vi "Splash Screen.vi"(8 "Error In":errorcluster) -> (0 "Error Out":errorcluster, 3 "Status":string)   [LabVIEW 2020]
doc: "This VI check for licensing and load Main program depending on license type."
uses:
  Control/State - Splash Screen.ctl
  Control/Page List Configuration.ctl
  <vilib>/Utility/sysdir.llb/System Directory Type.ctl
  <vilib>/Utility/miscctls.llb/LVPositionTypeDef.ctl
  <vilib>/picture/picture.llb/imagedata.ctl
  Control/License File Parameter.ctl
panel:
  in  "EXE Name":string="VSys Platform"
  out "Computer ID":string
  in  "stop":bool
  out "Version":string
  out "BG Image":picture
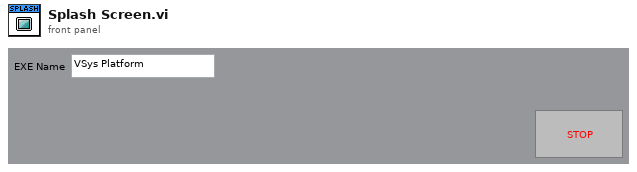
[diagram p1: front panel]
types:
  T1 = typedef "Page List Configuration.ctl" = cluster{"HMI Configuration":cluster{"EXE Name":string, "Project Name":string, "Max Page No":i32, "HMI State":enum32{"Invalid", "Standard", "Closed", "Hidden", "Minimized", "Maximized"}, "Version":enum16{"Demo", "User"}, "Check License":bool, "Font Size":u32, "Res: Height":i16, "Res: Width":i16, "License Level":enum16{"Level 1", "Level 2", "Level 3", "Level 4", "Level 5"}, "License Type":enum16{"Free", "Trial", "Subscription", "Perpetual"}}, "All HMI Module":string[], "Default HMI Module":string[], "Page Module":string[], "Page List: Level 1":string[], "Page List: Level 2":string[], "Page List: Level 3":string[], "All RT Module":string[], "Default RT Module":string[], "Acquire Enable Page":string[], "Log Enable Page":string[], "Run Page":string[], "Kill Page":string[], "Button":cluster{"Text":string[], "Tip Strip":string[]}}
  T2 = typedef "State - Splash Screen.ctl" = enum16{"Init", "Read Config", "Set BG Image", "Get Computer ID", "Check Licensing", "Load Main VI", "Close"}
  T3 = enum32{"Invalid", "Standard", "Closed", "Hidden", "Minimized", "Maximized"}
  T4 = typedef "LVPositionTypeDef.ctl" = cluster{"Left":i32, "Top":i32}
  T5 = enum16{"open", "replace", "create", "open or create", "replace or create", "replace or create with confirmation"}
  T6 = typedef "imagedata.ctl" = cluster{"image type":i32, "image depth":i32, "image":u8[], "mask":u8[], "colors":u32[], "Rectangle":cluster{"left":i16, "top":i16, "right":i16, "bottom":i16}}
  T7 = enum16{"Level 1", "Level 2", "Level 3", "Level 4", "Level 5"}
  T8 = typedef "License File Parameter.ctl" = cluster{"Expired Time":string, "Computer ID":string, "Product Name":string, "Period":i16, "Activated Time":string, "License Level":enum16{"Level 1", "Level 2", "Level 3", "Level 4", "Level 5"}, "License Type":enum16{"Free", "Trial", "Subscription", "Perpetual"}, "Log Time":string}
  T9 = enum32{"invalid app kind", "Development System", "Run Time System", "Student Edition", "Embedded LabVIEW", "Evaluation", "Custom"}
  T10 = typedef "System Directory Type.ctl" = i32
  T11 = enum16{"Free", "Trial", "Subscription", "Perpetual"}
  T12 = enum32{"Bad", "Idle", "Run top level", "Running"}
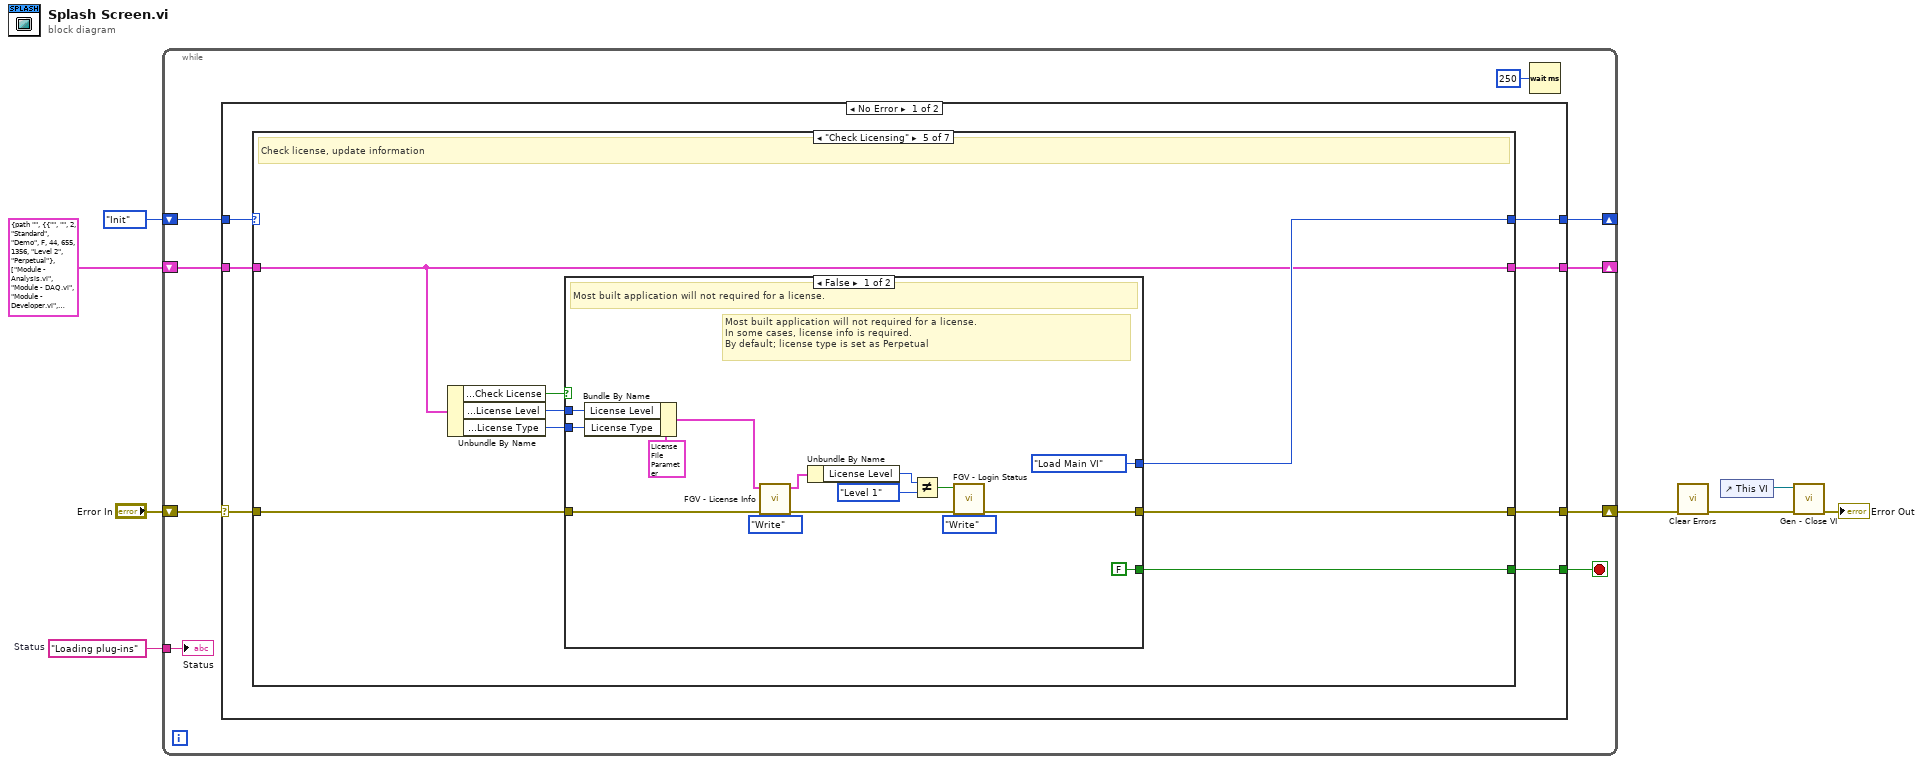
[diagram p0: block diagram]
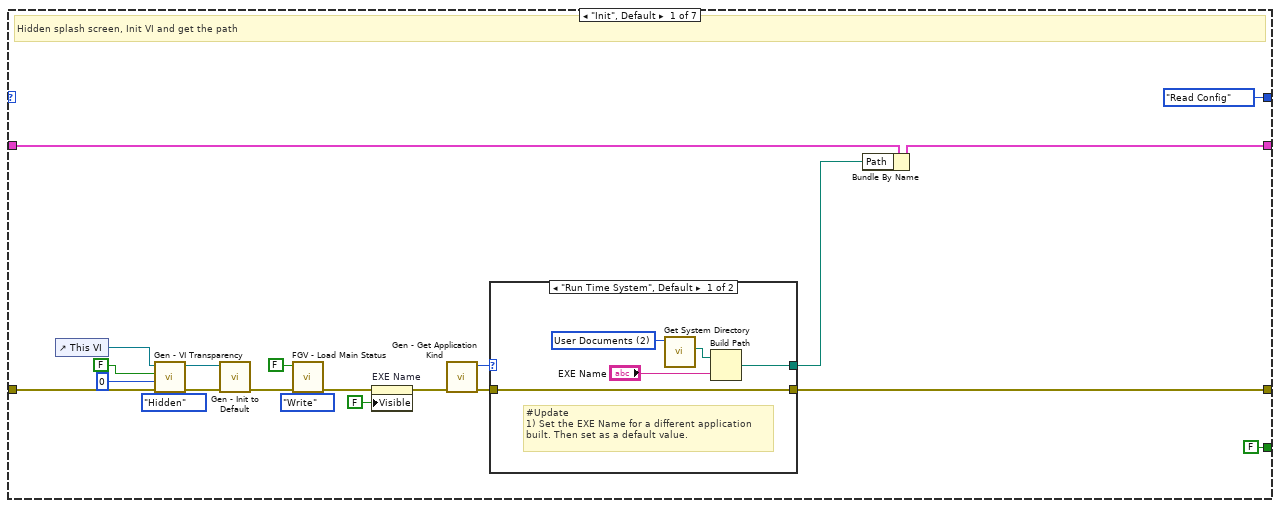
[diagram p2: hidden frame]
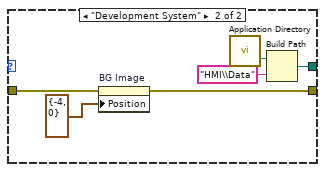
[diagram p3: hidden frame]
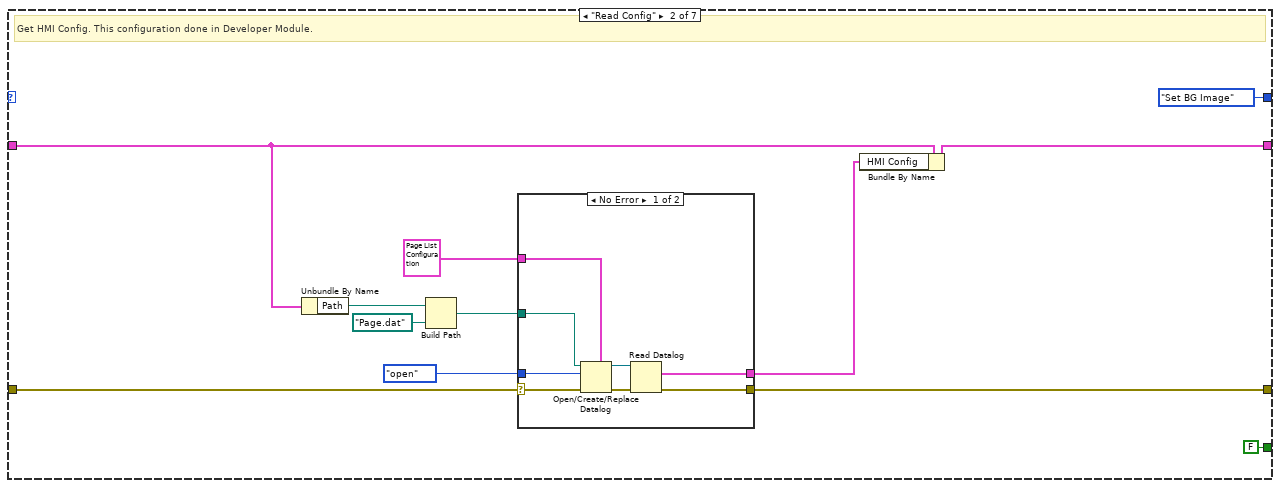
[diagram p4: hidden frame]
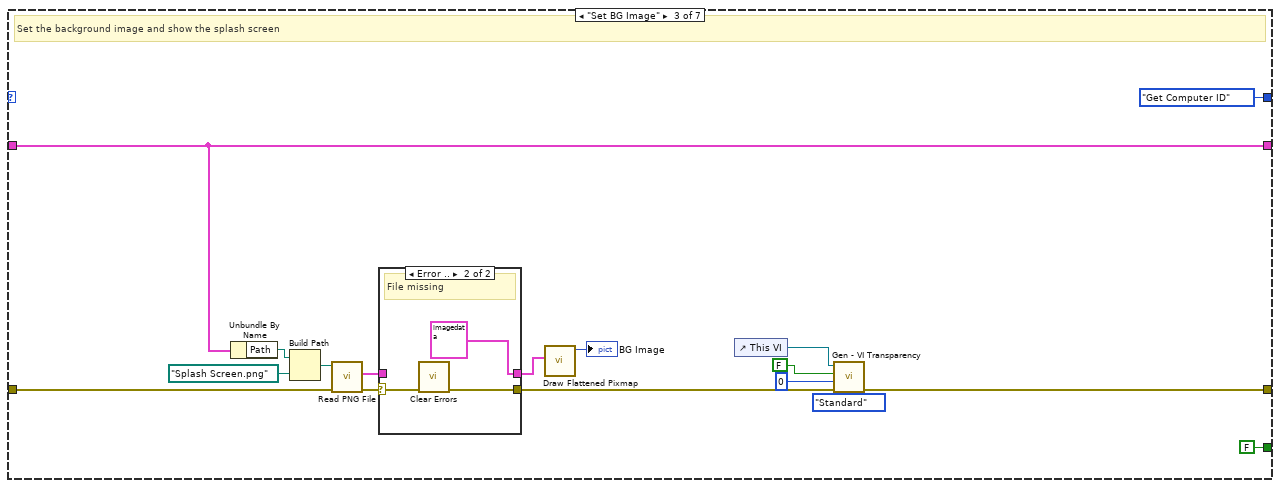
[diagram p6: hidden frame]
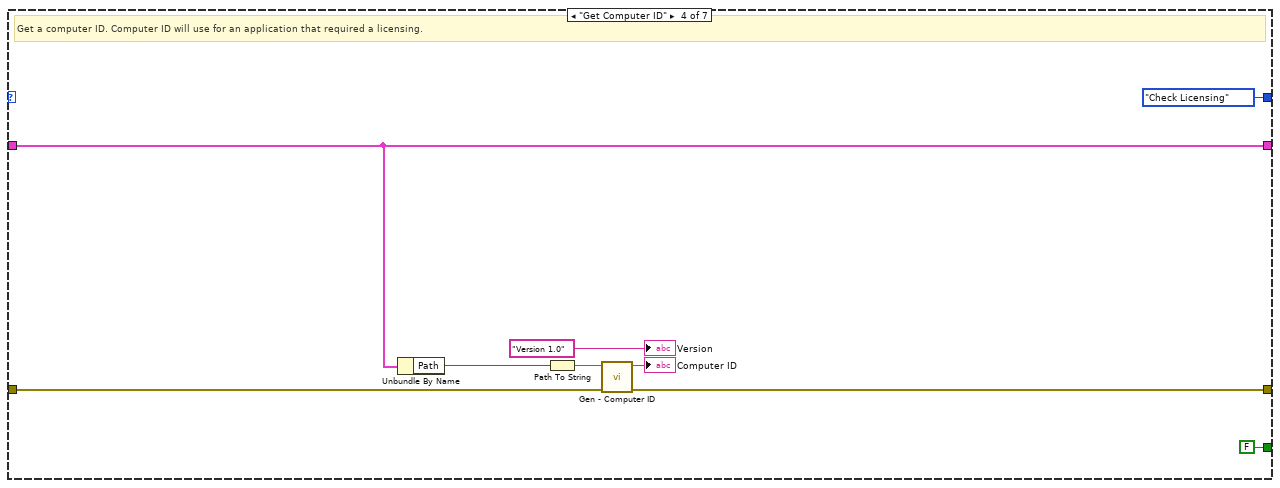
[diagram p8: hidden frame]
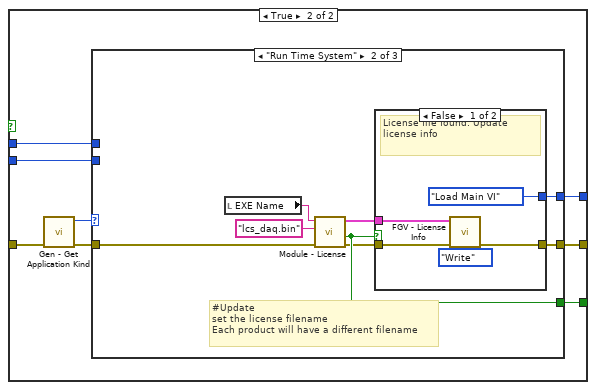
[diagram p9: hidden frame]
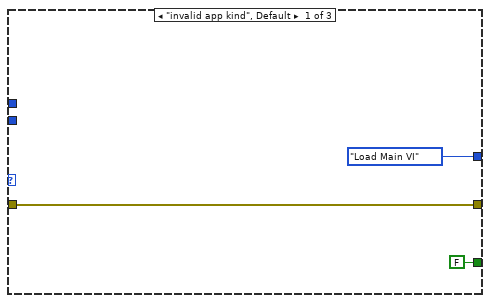
[diagram p10: hidden frame]
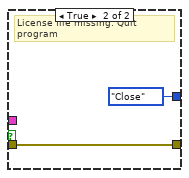
[diagram p11: hidden frame]
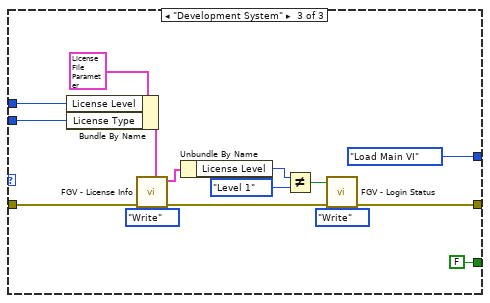
[diagram p12: hidden frame]
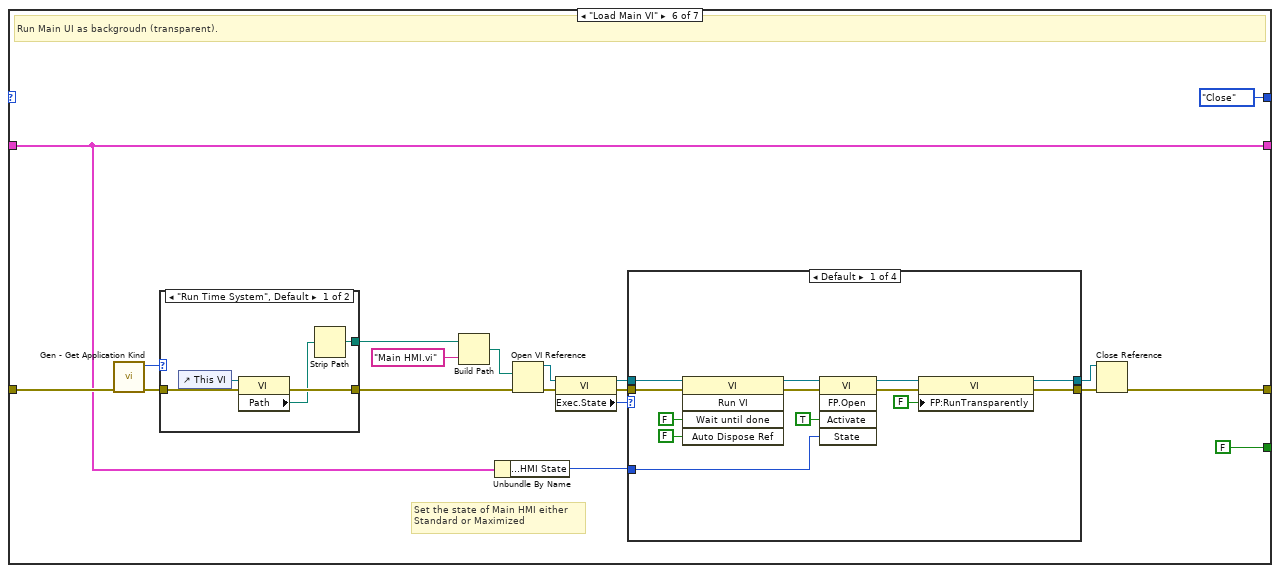
[diagram p13: hidden frame]
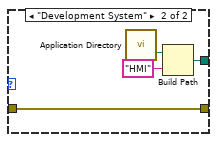
[diagram p14: hidden frame]
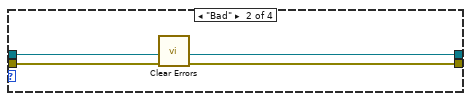
[diagram p15: hidden frame]
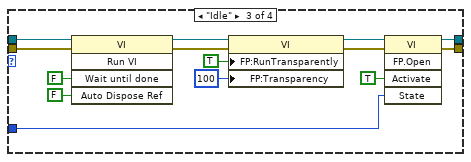
[diagram p16: hidden frame]
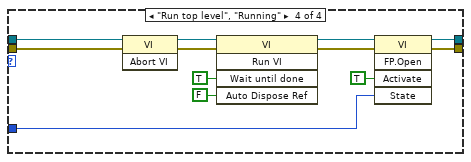
[diagram p17: hidden frame]
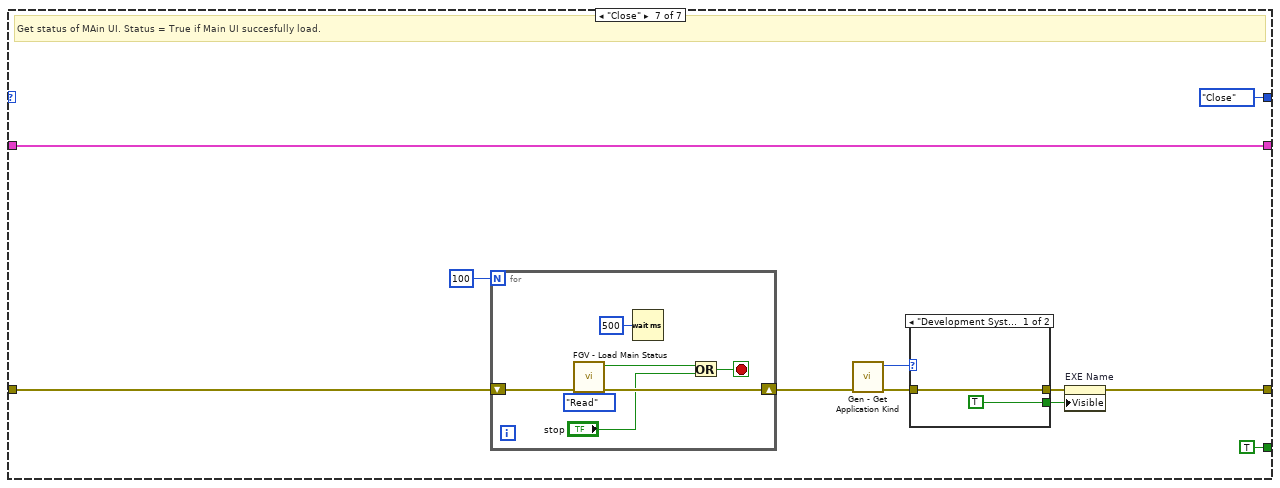
[diagram p18: hidden frame]
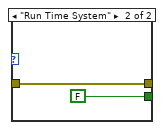
[diagram p19: hidden frame]
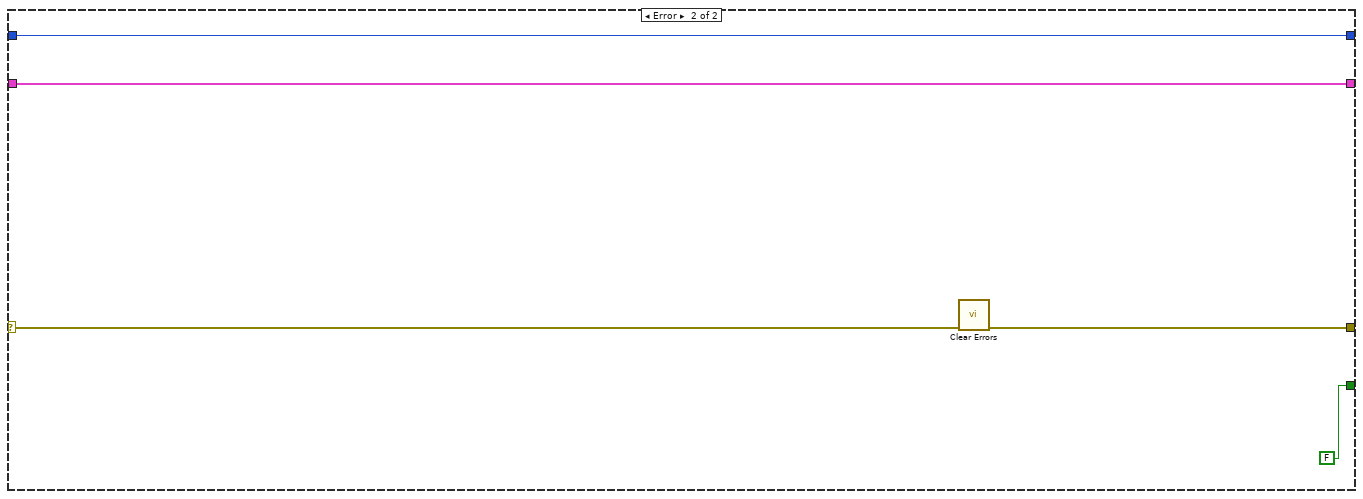
[diagram p20: hidden frame]
diagram:
  w7 = "Loading plug-ins"  # Status
  n1 = while {
    shift-right: [w16] -> w5
    shift-left: "Error In" -> [w17]
    shift-right: [w13] -> _
    shift-left: State_-_Splash_Screen."Init" ("State") -> [w15]
    tunnel: w7 -> [w11]
    shift-right: [w9] -> _
    shift-left: cluster{"Path":path, "HMI Config":T1} {"Path"=path "", "HMI Config"={"HMI Configuration"={"EXE Name"="", "Project Name"="", "Max Page No"=2, "HMI State"=enum."Standard", "Version"=enum."Demo", "Check License"=FALSE, "Font Size"=44, "Res: Height"=655, "Res: Width"=1356, "License Level"=enum."Level 2", "License Type"=enum."Perpetual"}, "All HMI Module"=["Module - Analysis.vi", "Module - DAQ.vi", "Module - Developer.vi", "Module - Error Management.vi", "Module - License.vi", "Module - Logging.vi", "Module - Network Stream PC.vi", "Module - NSV Comm PC.vi", "Module - Page Configuration.vi", "Module - Page Main.vi", "Module - Page Prediction.vi", "Module - Page Ranging.vi", "Module - Page User.vi", "Module - Template HMI - Copy.vi", "Module - Template HMI.vi", "Module - WebDAV.vi"], "Default HMI Module"=["Module - DAQ.vi", "Module - Network Stream PC.vi", "Module - NSV Comm PC.vi", "Module - Page Configuration.vi", "Module - Page Ranging.vi", "Module - Page Logging.vi", "Module - Analysis.vi", "Module - Page Prediction.vi"], "Page Module"=["Module - Page Configuration.vi", "Module - Page Ranging.vi", "Module - Analysis.vi", "Module - Page Prediction.vi"], "Page List: Level 1"=["Module - Page Main.vi", "Module - Page Device.vi", "Module - Page IO Setting.vi", "Module - Page Logging.vi", "Module - Page Scale.vi", "Module - Page Filter.vi", "Module - Page User.vi", "Module - Page Cloud.vi"], "Page List: Level 2"=["Module - Page Main.vi", "Module - Page Device.vi", "Module - Page IO Setting.vi", "Module - Page Logging.vi", "Module - Page Scale.vi", "Module - Page Filter.vi"], "Page List: Level 3"=["Module - Page Main.vi", "Module - Page Device.vi", "Module - Page IO Setting.vi"], "All RT Module"=[], "Default RT Module"=["Module - Page Configuration.vi", "Module - Page Main.vi"], "Acquire Enable Page"=["Module - Page Configuration.vi", "Module - Page Ranging.vi"], "Log Enable Page"=["Module - RT Device.vi", "Module - RT Git.vi"], "Run Page"=["Module - DAQmx AI.vi", "Module - DAQmx AO.vi", "Module - DAQmx DI.vi", "Module - DAQmx DO.vi"], "Kill Page"=["Module - Arduino DIO AI.vi"], "Button"={"Text"=["CONFIGURE", "RANGING", "ANALYSIS", "PREDICTION", "SCALE", "FILTER", "USER", "CLOUD", "ALARM", "Button 10", "Button 11", "Button 12", "Button 13", "Button 14", "Button 15"], "Tip Strip"=[]}}} -> [w10]
    stop <- w14 stop-if-true
    n2 = case shown="No Error" w17 {
      selector: w17 -> [w23 w270]
      tunnel: w15 -> [w22 w267]
      tunnel: [w24 w269] -> w16
      tunnel: [w21 FALSE] -> w14
      tunnel: [w20 w267] -> w13
      tunnel: w10 -> [w19 w266]
      tunnel: [w18 w266] -> w9
      frame No Error {
        n3 = case shown="\"Check Licensing\"" w22 {
          tunnel: [w26 w62 w79 w106 w117 w176 w248] -> w24
          tunnel: w23 -> [w41 w59 w90 w107 w114 w180 w254]
          tunnel: [FALSE FALSE FALSE ("License Missing?") FALSE ("License Missing?") w115 FALSE TRUE] -> w21
          tunnel: [State_-_Splash_Screen."Read Config" ("State") State_-_Splash_Screen."Set BG Image" ("State") State_-_Splash_Screen."Get Computer ID" ("State") State_-_Splash_Screen."Check Licensing" ("State") w116 State_-_Splash_Screen."Close" ("State") State_-_Splash_Screen."Close" ("State")] -> w20
          tunnel: w19 -> [w31 w61 w89 w105 w113 w175 w244]
          tunnel: [w27 w58 w89 w105 w113 w175 w244] -> w18
          frame "Init", Default {
            # "Hidden splash screen, Init VI and get the path"
            n4 = control-ref of="This VI"() -> (w43:refnum<vi>)
            n5 = call "Gen - VI Transparency.vi"("State"=T3."Hidden", "Error In"=w41, "Transparency"=u8 0, "Transparently?"=FALSE, "Ref VI"=w43) -> ("Error Out"=w42:errorcluster, "Ref VI Out"=w36:refnum<vi>)  [unwired: 5 in]
            n6 = call "Gen - Init to Default.vi"("Error in"=w42, "This VI"=w36) -> ("Error out"=w35:errorcluster)  [unwired: 8 in, 1 out]
            n7 = call "FGV - Load Main Status.vi"("Action"=enum16{"Read", "Write"}."Write", "Error In"=w35, "Status in"=FALSE) -> ("Error Out"=w33:errorcluster)  [unwired: 7 in, 1 out]
            n8 = property on="EXE Name" class="Str"(error in=w33, "Visible"=FALSE) -> (error out=w28:errorcluster)  [unwired: 1 in, 1 out]
            n9 = call "Gen - Get Application Kind.vi"("Error In"=w28) -> ("Error Out"=w29:errorcluster, "Application:Kind"=w30:T9)  [unwired: 9 in]
            n10 = case shown="\"Run Time System\", Default" w30 {
              tunnel: [w46 w54] -> w25
              tunnel: [w50 w52] -> w26
              tunnel: w29 -> [w50 w53]
              frame "Run Time System", Default {
                w47 = T10 2 items=["User Home"=0, "User Desktop"=1, "User Documents"=2, "User Application Data"=3, "User Preferences"=4, "User Temporary"=5, "Public Documents"=6, "Public Application Data"=7, "Public Preferences"=8, "Public Cache"=13, "System Core Libraries"=9, "System Installed Libraries"=10, "Application Files"=11, "Boot Volume Root"=12] ("system directory type")
                # "#Update\n1) Set the EXE Name for a different application \nbuilt. Then set as a default value."
                n11 = call <vilib>:"Get System Directory.vi"("system directory type"=w47) -> ("system directory"=w49:path)  [unwired: 10 in]
                n12 = Build Path(base path=w49, name or relative path="EXE Name") -> (appended path=w46:path)
              }
              frame "Development System" {
                n13 = property on="BG Image" class="Pict"(error in=w53, "Position"=T4 {"Left"=-4, "Top"=0}) -> (error out=w52:errorcluster)  [unwired: 1 in, 1 out]
                n14 = call <vilib>:"Application Directory.vi"() -> ("Application Directory"=w55:path)
                n15 = Build Path(base path=w55, name or relative path="HMI\\Data") -> (appended path=w54:path)
              }
            }
            n16 = Bundle By Name(cluster=w31, "Path"=w25) -> (w27:cluster{"Path":path, "HMI Config":T1})
          }
          frame "Read Config" {
            # "Get HMI Config. This configuration done in Developer Module."
            n17 = Unbundle By Name(w61) -> ("Path"=w60:path)
            n18 = Build Path(base path=w60, name or relative path=path "Page.dat") -> (appended path=w63:path)
            n19 = case shown="No Error" w59 {
              selector: w59 -> [w70 w78]
              tunnel: T1 {"HMI Configuration"={"EXE Name"="", "Project Name"="", "Max Page No"=2, "HMI State"=enum."Standard", "Version"=enum."Demo", "Check License"=FALSE, "Font Size"=44, "Res: Height"=655, "Res: Width"=1356, "License Level"=enum."Level 2", "License Type"=enum."Perpetual"}, "All HMI Module"=["Module - Analysis.vi", "Module - DAQ.vi", "Module - Developer.vi", "Module - Error Management.vi", "Module - License.vi", "Module - Logging.vi", "Module - Network Stream PC.vi", "Module - NSV Comm PC.vi", "Module - Page Configuration.vi", "Module - Page Main.vi", "Module - Page Prediction.vi", "Module - Page Ranging.vi", "Module - Page User.vi", "Module - Template HMI - Copy.vi", "Module - Template HMI.vi", "Module - WebDAV.vi"], "Default HMI Module"=["Module - DAQ.vi", "Module - Network Stream PC.vi", "Module - NSV Comm PC.vi", "Module - Page Configuration.vi", "Module - Page Ranging.vi", "Module - Page Logging.vi", "Module - Analysis.vi", "Module - Page Prediction.vi"], "Page Module"=["Module - Page Configuration.vi", "Module - Page Ranging.vi", "Module - Analysis.vi", "Module - Page Prediction.vi"], "Page List: Level 1"=["Module - Page Main.vi", "Module - Page Device.vi", "Module - Page IO Setting.vi", "Module - Page Logging.vi", "Module - Page Scale.vi", "Module - Page Filter.vi", "Module - Page User.vi", "Module - Page Cloud.vi"], "Page List: Level 2"=["Module - Page Main.vi", "Module - Page Device.vi", "Module - Page IO Setting.vi", "Module - Page Logging.vi", "Module - Page Scale.vi", "Module - Page Filter.vi"], "Page List: Level 3"=["Module - Page Main.vi", "Module - Page Device.vi", "Module - Page IO Setting.vi"], "All RT Module"=[], "Default RT Module"=["Module - Page Configuration.vi", "Module - Page Main.vi"], "Acquire Enable Page"=["Module - Page Configuration.vi", "Module - Page Ranging.vi"], "Log Enable Page"=["Module - RT Device.vi", "Module - RT Git.vi"], "Run Page"=["Module - DAQmx AI.vi", "Module - DAQmx AO.vi", "Module - DAQmx DI.vi", "Module - DAQmx DO.vi"], "Kill Page"=["Module - Arduino DIO AI.vi"], "Button"={"Text"=["CONFIGURE", "RANGING", "ANALYSIS", "PREDICTION", "SCALE", "FILTER", "USER", "CLOUD", "ALARM", "Button 10", "Button 11", "Button 12", "Button 13", "Button 14", "Button 15"], "Tip Strip"=[]}} ("Data Out 2") -> [w75 w77]
              tunnel: T5."open" ("operation (0:open)") -> [w74 _]
              tunnel: w63 -> [w73 _]
              tunnel: [w71 w78] -> w62
              tunnel: [w69 w77] -> w57
              frame No Error {
                n20 = Open/Create/Replace Datalog(5:w75, 8:w70, 10:w74, 11:w73) -> (0:w72:errorcluster, 3:w76:refnum<k1>)  [unwired: 2 in, 1 out]
                n21 = Read Datalog(4:w72, 7:w76) -> (0:w71:errorcluster, 2:w69:T1)  [unwired: 1 in, 1 out]
              }
              frame Error {
              }
            }
            n22 = Bundle By Name(cluster=w61, "HMI Config"=w57) -> (w58:cluster{"Path":path, "HMI Config":T1})
          }
          frame "Set BG Image" {
            # "Set the background image and show the splash screen"
            n23 = Unbundle By Name(w89) -> ("Path"=w88:path)
            n24 = Build Path(base path=w88, name or relative path=path "Splash Screen.png") -> (appended path=w93:path)
            n25 = call <vilib>:"Read PNG File.vi"("error in (no error)"=w90, "path to PNG file"=w93) -> ("error out"=w87:errorcluster, "image data"=w85:T6)  [unwired: 7 in, 1 out]
            n26 = case shown="Error .." w87 {
              selector: w87 -> [w97 w99]
              tunnel: [w97 w98] -> w86
              tunnel: [w96 T6 {"image type"=0, "image depth"=32, "image"=array[1013796 elements], "mask"=array[32184 elements], "colors"=[], "Rectangle"={"left"=0, "top"=0, "right"=567, "bottom"=447}} ("image data")] -> w84
              tunnel: w85 -> [w96 _]
              frame No Error {
              }
              frame Error {
                # "File missing"
                n27 = call <vilib>:"Clear Errors.vi"("error in (no error)"=w99) -> ("error out"=w98:errorcluster)  [unwired: 5 in, 1 out]
              }
            }
            n28 = call <vilib>:"Draw Flattened Pixmap.vi"("image data"=w84) -> ("new picture"=→"BG Image":picture)  [unwired: 8 in]
            n29 = control-ref of="This VI"() -> (w83:refnum<vi>)
            n30 = call "Gen - VI Transparency.vi"("State"=T3."Standard", "Error In"=w86, "Transparency"=u8 0, "Transparently?"=FALSE, "Ref VI"=w83) -> ("Error Out"=w79:errorcluster)  [unwired: 5 in, 1 out]
          }
          frame "Get Computer ID" {
            # "Get a computer ID. Computer ID will use for an application that required a licensing."
            n31 = Unbundle By Name(w105) -> ("Path"=w104:path)
            n32 = Path To String(path=w104) -> (string=w102:string)
            n33 = call "Gen - Computer ID.vi"("Error In"=w107, "Path"=w102) -> ("Error Out"=w106:errorcluster, "COMPUTER ID"=→"Computer ID":string)  [unwired: 8 in]
            "Version" <- "Version 1.0" ("Serial Number")
          }
          frame "Check Licensing" {
            # "Check license, update information"
            n34 = Unbundle By Name(w113) -> ("HMI Config.HMI Configuration.Check License"=w112:bool, "HMI Config.HMI Configuration.License Level"=w111:T7, "HMI Config.HMI Configuration.License Type"=w110:T11)
            n35 = case shown="False" w112 {
              tunnel: [w123 w140] -> w117
              tunnel: [State_-_Splash_Screen."Load Main VI" ("State") w139] -> w116
              tunnel: [FALSE ("License Missing?") w138] -> w115
              tunnel: w114 -> [w130 w137]
              tunnel: w111 -> [w119 w134]
              tunnel: w110 -> [w118 w133]
              frame False {
                # "Most built application will not required for a license. \nIn some cases, license info is required.\nBy default; license type is set as Perpetual"
                # "Most built application will not required for a license."
                n36 = Bundle By Name(cluster=T8 {"Expired Time"="", "Computer ID"="", "Product Name"="", "Period"=0, "Activated Time"="", "License Level"=enum."Level 1", "License Type"=enum."Perpetual", "Log Time"=""} ("License Info  In"), "License Level"=w119, "License Type"=w118) -> (w120:T8)
                n37 = call "FGV - License Info.vi"("FGV States"=enum16{"Read", "Write"}."Write", "Error In"=w130, "License Info  In"=w120) -> ("Error Out"=w126:errorcluster, "License Info"=w122:T8)  [unwired: 7 in]
                n38 = Unbundle By Name(w122) -> ("License Level"=w125:T7)
                n39 = Not Equal?(x=w125, y=T7."Level 1" ("License Level")) -> (x != y?=w121:bool)
                n40 = call "FGV - Login Status.vi"("Action"=enum16{"Read", "Write"}."Write", "Error In"=w126, "Login In"=w121) -> ("Error Out"=w123:errorcluster)  [unwired: 6 in, 2 out]
              }
              frame True {
                n41 = call "Gen - Get Application Kind.vi"("Error In"=w137) -> ("Error Out"=w136:errorcluster, "Application:Kind"=w135:T9)  [unwired: 9 in]
                n42 = case shown="\"Run Time System\"" w135 {
                  tunnel: w136 -> [w143 w151 w172]
                  tunnel: [w143 w150 w163] -> w140
                  tunnel: [State_-_Splash_Screen."Load Main VI" ("State") w149 State_-_Splash_Screen."Load Main VI" ("State")] -> w139
                  tunnel: [FALSE ("License Missing?") w148 FALSE ("License Missing?")] -> w138
                  tunnel: w134 -> [_ _ w160]
                  tunnel: w133 -> [_ _ w159]
                  frame "invalid app kind", Default {
                  }
                  frame "Run Time System" {
                    # "#Update\nset the license filename\nEach product will have a different filename"
                    n43 = local read "EXE Name"() -> (w144:string)
                    n44 = call "Module - License.vi"("Error In"=w151, "License Filename"="lcs_daq.bin", "Product Name"=w144) -> ("Error Out"=w147:errorcluster, "License Missing?"=w148:bool, "License Info"=w146:T8)  [unwired: 4 in, 2 out]
                    n45 = case shown="False" w148 {
                      tunnel: [w156 w157] -> w150
                      tunnel: [State_-_Splash_Screen."Load Main VI" ("State") State_-_Splash_Screen."Close" ("State")] -> w149
                      tunnel: w147 -> [w153 w157]
                      tunnel: w146 -> [w152 _]
                      frame False {
                        # "License file found. Update license info"
                        n46 = call "FGV - License Info.vi"("FGV States"=enum16{"Read", "Write"}."Write", "Error In"=w153, "License Info  In"=w152) -> ("Error Out"=w156:errorcluster)  [unwired: 7 in, 1 out]
                      }
                      frame True {
                        # "License file missing. Quit program"
                      }
                    }
                  }
                  frame "Development System" {
                    n47 = Bundle By Name(cluster=T8 {"Expired Time"="", "Computer ID"="", "Product Name"="", "Period"=0, "Activated Time"="", "License Level"=enum."Level 2", "License Type"=enum."Perpetual", "Log Time"=""} ("License Info  In"), "License Level"=w160, "License Type"=w159) -> (w161:T8)
                    n48 = call "FGV - License Info.vi"("FGV States"=enum16{"Read", "Write"}."Write", "Error In"=w172, "License Info  In"=w161) -> ("Error Out"=w164:errorcluster, "License Info"=w168:T8)  [unwired: 7 in]
                    n49 = Unbundle By Name(w168) -> ("License Level"=w167:T7)
                    n50 = Not Equal?(x=w167, y=T7."Level 1" ("License Level")) -> (x != y?=w165:bool)
                    n51 = call "FGV - Login Status.vi"("Action"=enum16{"Read", "Write"}."Write", "Error In"=w164, "Login In"=w165) -> ("Error Out"=w163:errorcluster)  [unwired: 6 in, 2 out]
                  }
                }
              }
            }
          }
          frame "Load Main VI" {
            # "Set the state of Main HMI either \nStandard or Maximized"
            # "Run Main UI as backgroudn (transparent)."
            n52 = call "Gen - Get Application Kind.vi"("Error In"=w180) -> ("Error Out"=w179:errorcluster, "Application:Kind"=w181:T9)  [unwired: 9 in]
            n53 = case shown="\"Run Time System\", Default" w181 {
              tunnel: [w193 w198] -> w185
              tunnel: [w196 w201] -> w182
              tunnel: w179 -> [w195 w201]
              frame "Run Time System", Default {
                n54 = control-ref of="This VI"() -> (w197:refnum<vi>)
                n55 = property class="VI"(reference=w197, error in=w195) -> (error out=w196:errorcluster, "Path"=w194:path)  [unwired: 1 out]
                n56 = Strip Path(path=w194) -> (stripped path=w193:path)  [unwired: 1 out]
              }
              frame "Development System" {
                n57 = call <vilib>:"Application Directory.vi"() -> ("Application Directory"=w199:path)
                n58 = Build Path(base path=w199, name or relative path="HMI") -> (appended path=w198:path)
              }
            }
            n59 = Build Path(base path=w185, name or relative path="Main HMI.vi") -> (appended path=w183:path)
            n60 = Unbundle By Name(w175) -> ("HMI Config.HMI Configuration.HMI State"=w174:T3)
            n61 = Open VI Reference(vi path=w183, error in (no error)=w182) -> (vi reference=w188:refnum<vi>, error out=w187:errorcluster)  [unwired: 4 in]
            n62 = property class="VI"(reference=w188, error in=w187) -> (reference out=w190:refnum<vi>, error out=w189:errorcluster, "Exec.State"=w191:T12)
            n63 = case shown="Default" w191 {
              tunnel: w189 -> [w212 w217 w229 w243]
              tunnel: w190 -> [w211 w216 w228 w242]
              tunnel: [w206 w216 w226 w234] -> w178
              tunnel: [w205 w215 w225 w233] -> w177
              tunnel: w174 -> [w202 _ w218 w232]
              frame Default {
                n64 = invoke class="VI" method="Run VI"(reference=w211, error in=w212, "Wait until done"=FALSE ("Wait Until Done"), "Auto Dispose Ref"=FALSE ("Auto Dispose Reference")) -> (reference out=w209:refnum<vi>, error out=w210:errorcluster)  [unwired: 1 in, 3 out]
                n65 = invoke class="VI" method="FP.Open"(reference=w209, error in=w210, "Activate"=TRUE ("Activate?"), "State"=w202) -> (reference out=w207:refnum<vi>, error out=w204:errorcluster)  [unwired: 1 in, 3 out]
                n66 = property class="VI"(reference=w207, error in=w204, "FP:RunTransparently"=FALSE ("Front Panel Window:Run VI Transparently")) -> (reference out=w206:refnum<vi>, error out=w205:errorcluster)
              }
              frame "Bad" {
                n67 = call <vilib>:"Clear Errors.vi"("error in (no error)"=w217) -> ("error out"=w215:errorcluster)  [unwired: 5 in, 1 out]
              }
              frame "Idle" {
                n68 = invoke class="VI" method="Run VI"(reference=w228, error in=w229, "Wait until done"=FALSE ("Wait Until Done"), "Auto Dispose Ref"=FALSE ("Auto Dispose Reference")) -> (reference out=w221:refnum<vi>, error out=w223:errorcluster)  [unwired: 1 in, 3 out]
                n69 = property class="VI"(reference=w221, error in=w223, "FP:RunTransparently"=TRUE ("Front Panel Window:Run VI Transparently"), "FP:Transparency"=u8 100 ("Front Panel Window:Transparency")) -> (reference out=w220:refnum<vi>, error out=w222:errorcluster)
                n70 = invoke class="VI" method="FP.Open"(reference=w220, error in=w222, "Activate"=TRUE ("Activate?"), "State"=w218) -> (reference out=w226:refnum<vi>, error out=w225:errorcluster)  [unwired: 1 in, 3 out]
              }
              frame "Run top level", "Running" {
                n71 = invoke class="VI" method="Abort VI"(reference=w242, error in=w243) -> (reference out=w238:refnum<vi>, error out=w239:errorcluster)  [unwired: 1 in, 1 out]
                n72 = invoke class="VI" method="Run VI"(reference=w238, error in=w239, "Wait until done"=TRUE ("Wait Until Done"), "Auto Dispose Ref"=FALSE ("Auto Dispose Reference")) -> (reference out=w236:refnum<vi>, error out=w235:errorcluster)  [unwired: 1 in, 3 out]
                n73 = invoke class="VI" method="FP.Open"(reference=w236, error in=w235, "Activate"=TRUE ("Activate?"), "State"=w232) -> (reference out=w234:refnum<vi>, error out=w233:errorcluster)  [unwired: 1 in, 3 out]
              }
            }
            n74 = Close Reference(reference=w178, error in (no error)=w177) -> (error out=w176:errorcluster)
          }
          frame "Close" {
            # "Get status of MAin UI. Status = True if Main UI succesfully load."
            n75 = for {
              N: 100 -> [_]
              shift-right: [w264] -> w249
              shift-left: w254 -> [w265]
              stop <- w259 stop-if-true
              n76 = call "FGV - Load Main Status.vi"("Action"=enum16{"Read", "Write"}."Read", "Error In"=w265) -> ("Error Out"=w264:errorcluster, "Status Out"=w261:bool)  [unwired: 8 in]
              n77 = Wait (ms)(milliseconds to wait=u32 500) -> ()  [unwired: 1 out]
              n78 = Or(x=w261, y="stop") -> (x .or. y?=w259:bool)
            }
            n79 = call "Gen - Get Application Kind.vi"("Error In"=w249) -> ("Error Out"=w245:errorcluster, "Application:Kind"=w247:T9)  [unwired: 9 in]
            n80 = case shown="\"Development System\", Default" w247 {
              tunnel: [TRUE ("Visible") FALSE ("Visible")] -> w250
              tunnel: [w256 w258] -> w246
              tunnel: w245 -> [w256 w258]
              frame "Development System", Default {
              }
              frame "Run Time System" {
              }
            }
            n81 = property on="EXE Name" class="Str"(error in=w246, "Visible"=w250) -> (error out=w248:errorcluster)  [unwired: 1 in, 1 out]
          }
        }
      }
      frame Error {
        n82 = call <vilib>:"Clear Errors.vi"("error in (no error)"=w270) -> ("error out"=w269:errorcluster)  [unwired: 5 in, 1 out]
      }
    }
    n83 = Wait (ms)(milliseconds to wait=u32 250) -> ()  [unwired: 1 out]
    "Status" <- w11
  }
  n84 = call <vilib>:"Clear Errors.vi"("error in (no error)"=w5) -> ("error out"=w3:errorcluster)  [unwired: 5 in, 1 out]
  n85 = control-ref of="This VI"() -> (w6:refnum<vi>)
  n86 = call "Gen - Close VI.vi"("Error In"=w3, "Ref VI"=w6) -> ("Error Out"=→"Error Out":errorcluster)  [unwired: 9 in]
